vi "查询数据库.vi"() -> (2 "数据":string[][](array[string]))   [LabVIEW 2015]
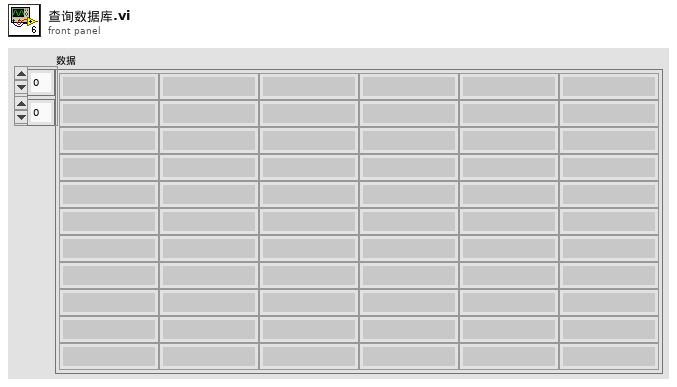
[diagram p1: front panel]
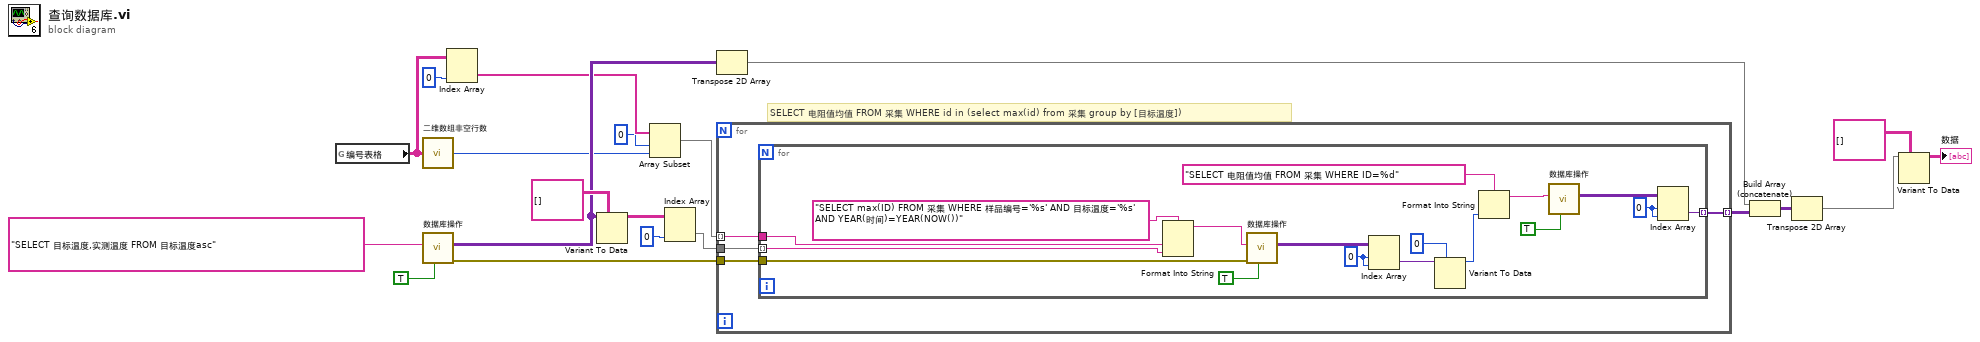
[diagram p0: block diagram]
diagram:
  # "SELECT 电阻值均值 FROM 采集 WHERE id in (select max(id) from 采集 group by [目标温度])"
  n1 = global read "全局.vi" "编号表格"() -> (w6:string[][])
  n2 = call "二维数组非空行数.vi"("数组"=w6) -> ("行数"=w3:i32)
  n3 = call "数据库操作.vi"("返回数据"=TRUE, "SQL query"="SELECT 目标温度,实测温度 FROM 目标温度asc" ("SQL")) -> ("error out"=w19:errorcluster, "recordset data"=w12:variant[][])  [unwired: 8 in]
  n4 = Index Array(array=w6, index (col)=0 ("禁用的索引 (列)")) -> (element=w5:string[])  [unwired: 1 in]
  n5 = Variant To Data(type=string[][] [], Variant=w12) -> (data=w10:string[][])  [unwired: 1 in, 1 out]
  n6 = Array Subset(array=w5, index=0 ("索引"), length=w3) -> (w2:string[])
  n7 = Index Array(array=w10, index (col)=0 ("禁用的索引 (列)")) -> (element=w9:string[])  [unwired: 1 in]
  n8 = Transpose 2D Array(2D array=w12) -> (transposed array=w18:variant[][])
  n9 = for {
    tunnel: w2 -> [w24] mode=indexing
    tunnel: w19 -> [w23]
    tunnel: w9 -> [w22]
    tunnel: [w21] -> w8 mode=indexing
    n10 = for {
      tunnel: [w26] -> w21 mode=indexing
      tunnel: w24 -> [w38]
      tunnel: w23 -> [w37]
      tunnel: w22 -> [w36] mode=indexing
      w27 = 0 ("索引 (行)")
      w34 = 0 ("索引 (行)")
      n11 = Format Into String(format string="SELECT max(ID) FROM 采集 WHERE 样品编号='%s' AND 目标温度='%s' AND YEAR(时间)=YEAR(NOW())" ("SQL"), w38, w36) -> (resulting string=w40:string)  [unwired: 2 in, 1 out]
      n12 = call "数据库操作.vi"("返回数据"=TRUE, "error in (no error)"=w37, "SQL query"=w40) -> ("recordset data"=w35:variant[][])  [unwired: 7 in, 1 out]
      n13 = Index Array(array=w35, index (row)=w34, index (col)=w34) -> (element=w32:variant)
      n14 = Variant To Data(type=0, Variant=w32) -> (data=w31:i32)  [unwired: 1 in, 1 out]
      n15 = Format Into String(format string="SELECT 电阻值均值 FROM 采集 WHERE ID=%d" ("SQL"), w31) -> (resulting string=w30:string)  [unwired: 2 in, 1 out]
      n16 = call "数据库操作.vi"("返回数据"=TRUE, "SQL query"=w30) -> ("recordset data"=w28:variant[][])  [unwired: 8 in, 1 out]
      n17 = Index Array(array=w28, index (row)=w27, index (col)=w27) -> (element=w26:variant)
    }
  }
  n18 = Build Array (concatenate)(w18, w8) -> (w17:variant[][])
  n19 = Transpose 2D Array(2D array=w17) -> (transposed array=w16:variant[][])
  n20 = Variant To Data(type=string[][] [], Variant=w16) -> (data=→"数据":string[][])  [unwired: 1 in, 1 out]
